vi "Export_Waveforms.vi"() -> ()   [LabVIEW 2011]
uses:
  <vilib>/express/express analysis/Spectral/Block/exnSpectralBlock spectral measurements power poly.vi
  <vilib>/express/express analysis/Spectral/Block/exnSpectralBlock spectral measurements power WFM.vi
  <vilib>/express/express analysis/Spectral/XNode/ExpressSpectralMeasurementsBlockNode.xnode
panel:
  out "appended path":path
  in  "header? (write header:T)":bool=TRUE
  in  "multiple columns? (single:F)":bool
  in  "Steps":i32
  out "Waveform Graph 2":waveform(dbl)[](graph)
  out "spectral Graph":cluster{"f0":dbl, "df":dbl, "magnitude":dbl[]}[](graph)
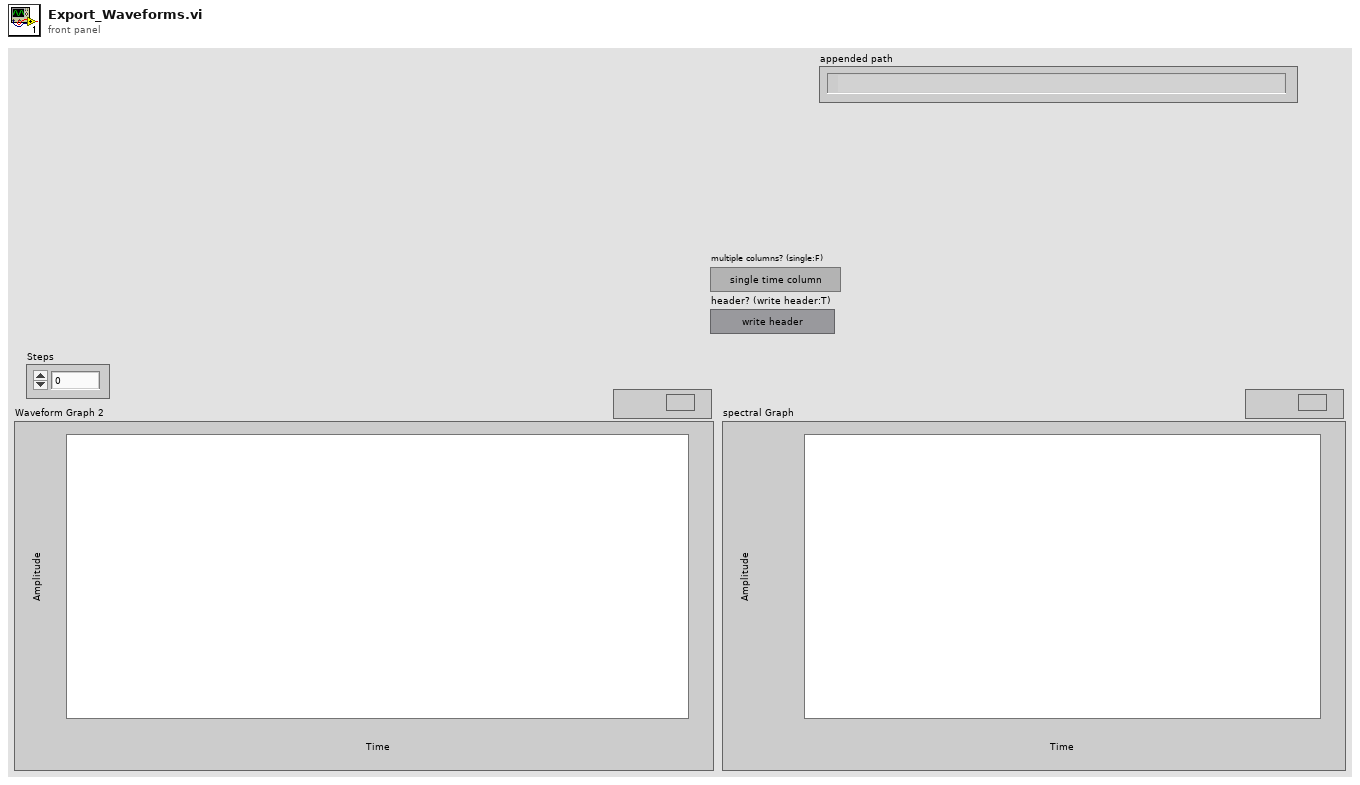
[diagram p1: front panel]
types:
  T1 = enum16{"open", "replace", "create", "open or create", "replace or create", "replace or create with confirmation"}
  T2 = cluster{"averaging mode":u16, "weighting mode":u16, "number of averages":u32}
  T3 = cluster{"dB On (F)":bool, "unwrap phase (F)":bool, "convert to degree (F)":bool}
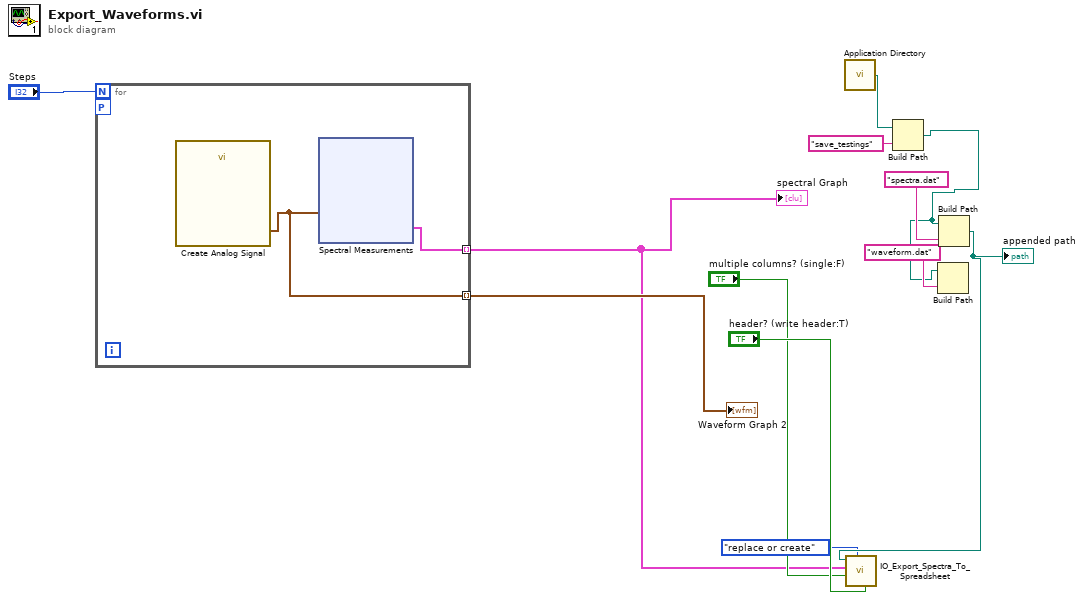
[diagram p0: block diagram]
diagram:
  n1 = for {
    N: "Steps" -> [_]
    workers-P: _ -> [_]
    tunnel: [w14] -> w6 mode=indexing
    tunnel: [w13] -> w9 mode=indexing
    n2 = call "Create Analog Signal"() -> ("white gaussian noise"=w13:waveform(dbl))  [unwired: 18 in, 1 out]
    n3 = xnode "Spectral Measurements"("Signals"=w13) -> ("Power Spectrum"=w14:cluster{"f0":dbl, "df":dbl, "magnitude":dbl[]})  [unwired: 1 in, 1 out]
  }
  "spectral Graph" <- w6
  "Waveform Graph 2" <- w9
  n4 = call <vilib>:"Application Directory.vi"() -> ("Application Directory"=w2:path)
  n5 = Build Path(base path=w2, name or relative path="save_testings") -> (appended path=w3:path)
  n6 = Build Path(base path=w3, name or relative path="waveform.dat") -> ()  [unwired: 1 out]
  n7 = Build Path(base path=w3, name or relative path="spectra.dat") -> (appended path=w5:path)
  "appended path" <- w5
  n8 = call "IO_Export_Spectra_To_Spreadsheet.vi"("header? (write header:T)"="header? (write header:T)", "operation (0:open)"=T1."replace or create", "multiple time columns? (single:F)"="multiple columns? (single:F)", "Array 2"=w6, "file path (dialog if empty)"=w5) -> ()  [unwired: 7 in]
